vi "Write AppOutputData.vi"(8 "error in (no error)":errorcluster, 10 "AppOutputData":variant, 11 "AppPluginsBase in":refnum<class "AppPluginsBase.lvclass">) -> (0 "error out":errorcluster, 3 "AppPluginsBase out":refnum<class "AppPluginsBase.lvclass">)   [LabVIEW 2017, in "AppPlugins.lvlib" / "AppPluginsBase.lvclass"]
uses:
  AppPluginsBase.lvclass
  AppPluginsBase.lvclass/AppPluginsBase.ctl
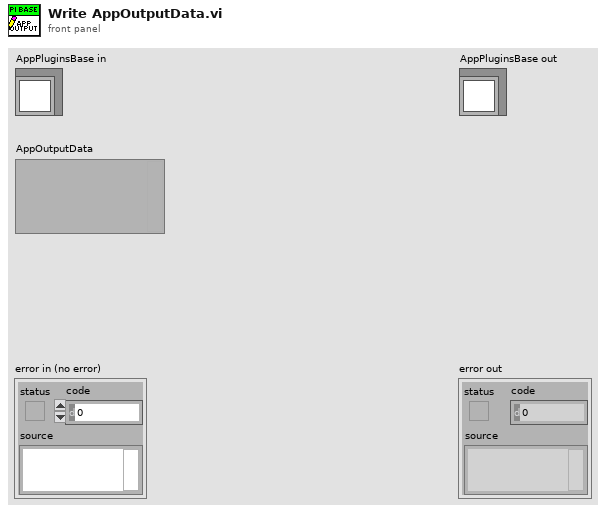
[diagram p1: front panel]
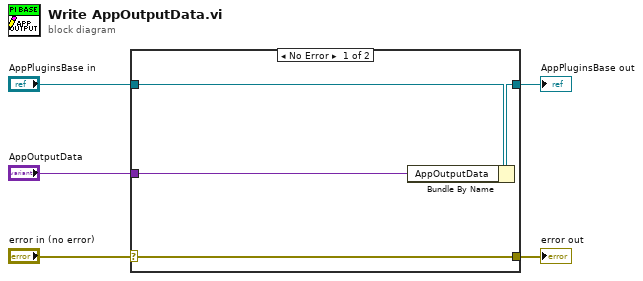
[diagram p0: block diagram]
diagram:
  n1 = case shown="No Error" "error in (no error)" {
    selector: "error in (no error)" -> [w9 w10]
    tunnel: [w9 w10] -> w4
    tunnel: [w7 w11] -> w2
    tunnel: "AppPluginsBase in" -> [w8 w11]
    tunnel: "AppOutputData" -> [w6 _]
    frame No Error {
      n2 = Bundle By Name(cluster=w8, "AppOutputData"=w6) -> (w7:refnum<class "AppPluginsBase.lvclass">)
    }
    frame Error {
    }
  }
  "error out" <- w4
  "AppPluginsBase out" <- w2
